vi "RealIO.vi"(10 "AllControls Out":T1) -> ()   [LabVIEW 2017]
uses:
  Ctrls/AllControls.ctl
  Ctrls/AlarmIndex.ctl
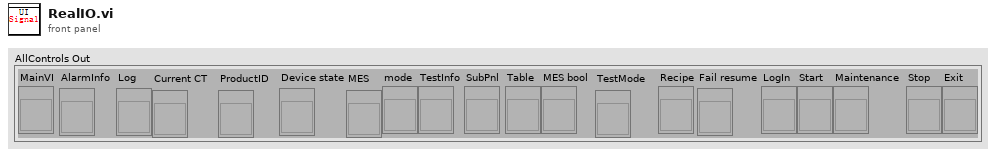
[diagram p1: front panel]
types:
  T1 = typedef "AllControls.ctl" = cluster{"MainVI":refnum<vi>, "AlarmInfo":refnum<vi>, "Log":refnum<vi>, "Current CT":refnum<vi>, "ProductID":refnum<vi>, "Device state":refnum<vi>, "MES":refnum<vi>, "mode":refnum<vi>, "TestInfo":refnum<vi>, "SubPnl":refnum<vi>, "Table":refnum<vi>, "MES bool":refnum<vi>, "TestMode":refnum<vi>, "Recipe":refnum<vi>, "Fail resume":refnum<vi>, "LogIn":refnum<vi>, "Start":refnum<vi>, "Maintenance":refnum<vi>, "Stop":refnum<vi>, "Exit":refnum<vi>}
  T2 = typedef "AlarmIndex.ctl" = enum16{"E-Stop", "Safety light grid", "UUT Sealing Cylinder HomePoint", "UUT Sealing Cylinder WorkPoint", "Orifice fixed Cylinder L HomePoint", "Orifice fixed Cylinder L WorkPoint", "Orifice fixed Cylinder R HomePoint", "Orifice fixed Cylinder R WorkPoint", "UUT Cylinder HomePoint", "UUT Cylinder WorkPoint", "Carrier fixed Cylinder L HomePoint", "Carrier fixed Cylinder L WorkPoint", "Carrier fixed Cylinder R HomePoint", "Carrier fixed Cylinder R WorkPoint", "Probe Cylinder HomePoint", "Probe Cylinder WorkPoint", "Motor Error", "Test Error"}
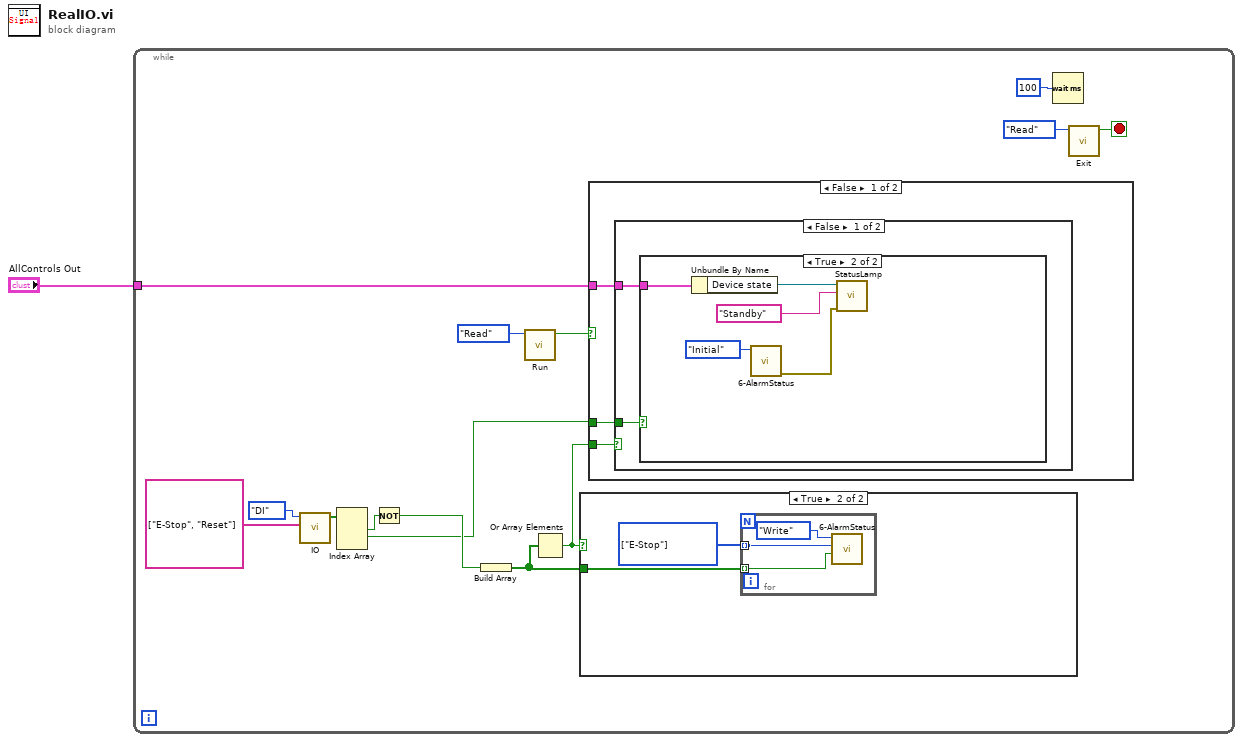
[diagram p0: block diagram]
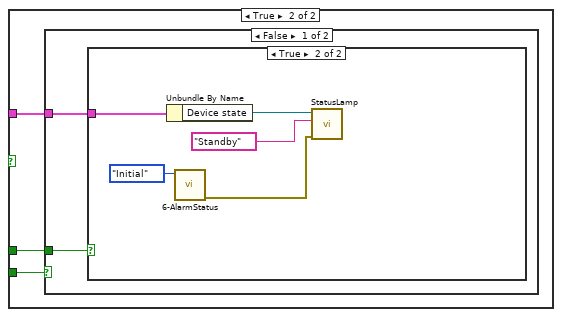
[diagram p5: hidden frame]
diagram:
  n1 = while {
    tunnel: "AllControls Out" -> [w6]
    stop <- w15 stop-if-true
    n2 = call "IO.vi"("IO Name"=string[] ["E-Stop", "Reset"], "IO?"=enum16{"DI", "DO"}."DI") -> ("DI"=w9:bool[])  [unwired: 8 in, 1 out]
    n3 = Index Array(array=w9) -> (element #1=w10:bool, element #2=w2:bool)  [unwired: 3 in, 1 out]
    n4 = Not(x=w10) -> (.not. x?=w3:bool)
    n5 = Build Array(w3) -> (w5:bool[])
    n6 = call "Run.vi"("Step"=enum16{"Initial", "Write", "Read"}."Read") -> ("Run Out"=w7:bool)  [unwired: 9 in, 1 out]
    n7 = Or Array Elements(Boolean array=w5) -> (logical OR=w4:bool)
    n8 = case shown="True" w4 {
      tunnel: w5 -> [_ w17]
      frame False {
      }
      frame True {
        w16 = T2[] [enum."E-Stop"] items=["E-Stop", "Safety light grid", "UUT Sealing Cylinder HomePoint", "UUT Sealing Cylinder WorkPoint", "Orifice fixed Cylinder L HomePoint", "Orifice fixed Cylinder L WorkPoint", "Orifice fixed Cylinder R HomePoint", "Orifice fixed Cylinder R WorkPoint", "UUT Cylinder HomePoint", "UUT Cylinder WorkPoint", "Carrier fixed Cylinder L HomePoint", "Carrier fixed Cylinder L WorkPoint", "Carrier fixed Cylinder R HomePoint", "Carrier fixed Cylinder R WorkPoint", "Probe Cylinder HomePoint", "Probe Cylinder WorkPoint", "Motor Error", "Test Error"]
        n9 = for {
          tunnel: w16 -> [w20] mode=indexing
          tunnel: w17 -> [w18] mode=indexing
          n10 = call "6-AlarmStatus.vi"("AlarmValue"=w18, "AlarmIndex"=w20, "Step"=enum16{"Initial", "Write", "Read"}."Write") -> ()  [unwired: 7 in, 2 out]
        }
      }
    }
    n11 = case shown="False" w7 {
      tunnel: w2 -> [w23 w32]
      tunnel: w6 -> [w22 w31]
      tunnel: w4 -> [w21 w33]
      frame False {
        n12 = case shown="False" w21 {
          tunnel: w23 -> [w25 _]
          tunnel: w22 -> [w24 _]
          frame False {
            n13 = case shown="True" w25 {
              tunnel: w24 -> [_ w29]
              frame False {
              }
              frame True {
                n14 = Unbundle By Name(w29) -> ("Device state"=w30:refnum<vi>)
                n15 = call "6-AlarmStatus.vi"("Step"=enum16{"Initial", "Write", "Read"}."Initial") -> ("error out"=w26:errorcluster)  [unwired: 9 in, 1 out]
                n16 = call "StatusLamp.vi"("错误输入（无错误）"=w26, "State"="Standby", "Boolean输入"=w30) -> ()  [unwired: 8 in, 1 out]
              }
            }
          }
          frame True {
          }
        }
      }
      frame True {
        n17 = case shown="False" w33 {
          tunnel: w32 -> [w35 _]
          tunnel: w31 -> [w34 _]
          frame False {
            n18 = case shown="True" w35 {
              tunnel: w34 -> [_ w37]
              frame False {
              }
              frame True {
                n19 = Unbundle By Name(w37) -> ("Device state"=w39:refnum<vi>)
                n20 = call "6-AlarmStatus.vi"("Step"=enum16{"Initial", "Write", "Read"}."Initial") -> ("error out"=w36:errorcluster)  [unwired: 9 in, 1 out]
                n21 = call "StatusLamp.vi"("错误输入（无错误）"=w36, "State"="Standby", "Boolean输入"=w39) -> ()  [unwired: 8 in, 1 out]
              }
            }
          }
          frame True {
          }
        }
      }
    }
    n22 = Wait (ms)(milliseconds to wait=u32 100 ("等待时间（毫秒）")) -> ()  [unwired: 1 out]
    n23 = call "Exit.vi"("Step"=enum16{"Initial", "Write", "Read"}."Read") -> ("Exit Out"=w15:bool)  [unwired: 9 in, 1 out]
  }
